vi "cno_isisubopt.vi"(0 "P":dbl[](array[numeric]), 1 "cno data":T5, 3 "tuning parameters":T1={"constraint weight"=1.0, "maximum minor iterations"=10}, 5 "L":dbl[](array[numeric]), 7 "H":dbl[][](array[numeric]), 9 "OB":dbl[](array[numeric]), 11 "error in (no error)":errorcluster, 12 "PB":dbl[][](array[numeric]), 14 "user defined functions":T2) -> (4 "P":dbl[](array[numeric]), 6 "L":dbl[](array[numeric]), 8 "H":dbl[][](array[numeric]), 10 "number of function calls":i32, 15 "error out":errorcluster)   [LabVIEW 2014, in "NI_Gmath.lvlib"]
uses:
  NI_Gmath.lvlib
  cno_data.ctl
  cno_user defined functions.ctl
  cno_user objective function ref.ctl
  objective function data.ctl
  cno_tuning parameters.ctl
  fpuIEEE64_finiteDiffConstants.ctl
  Real Outer Product.vi
  Real Cholesky Factorization.vi
  A x Vector.vi
  Real A x B.vi
  Full Cholesky Factorization.vi
  Full Real Matrix Cholesky Factorization.vi
  Create Special Real Matrix.vi
  Matrix To Array - RM.vi
  Real Inverse Matrix.vi
  Matrix left divisionMV.vi
  NI_AALBase.lvlib
  NI_AALPro.lvlib
  NI_Matrix.lvlib
panel:
  out "B":dbl[](array[numeric])
  out "G":dbl[](array[numeric])
  out "A":dbl[][](array[numeric])
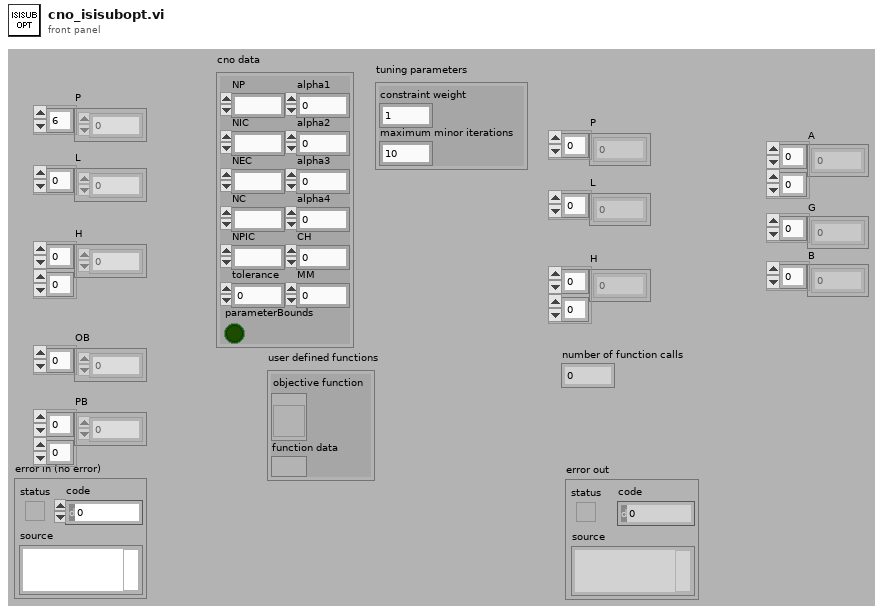
[diagram p1: front panel]
types:
  T1 = typedef "NI_Gmath.lvlib/cno_tuning parameters.ctl" = cluster{"constraint weight":dbl, "maximum minor iterations":i32}
  T2 = typedef "NI_Gmath.lvlib/cno_user defined functions.ctl" = cluster{"objective function":T3, "function data":T4}
  T3 = typedef "NI_Gmath.lvlib/cno_user objective function ref.ctl" = refnum<vi>
  T4 = typedef "NI_Gmath.lvlib/objective function data.ctl" = variant
  T5 = typedef "NI_Gmath.lvlib/cno_data.ctl" = cluster{"NP":i32, "NIC":i32, "NEC":i32, "NC":i32, "NPIC":i32, "parameterBounds":bool, "alpha1":dbl, "alpha2":dbl, "alpha3":dbl, "alpha4":dbl, "CH":i32, "MM":i32, "tolerance":dbl}
  T6 = enum32{"General", "Positive Definite", "Lower Triangular", "Upper Triangular"}
  T7 = enum32{"Identity", "Diagonal", "Toepliz", "Vandermonde", "Companion"}
  T8 = typedef "NI_Gmath.lvlib/fpuIEEE64_finiteDiffConstants.ctl" = dbl
  T9 = typedef "NI_Matrix.lvlib/RealMatrix.ctl" = dbl[][]
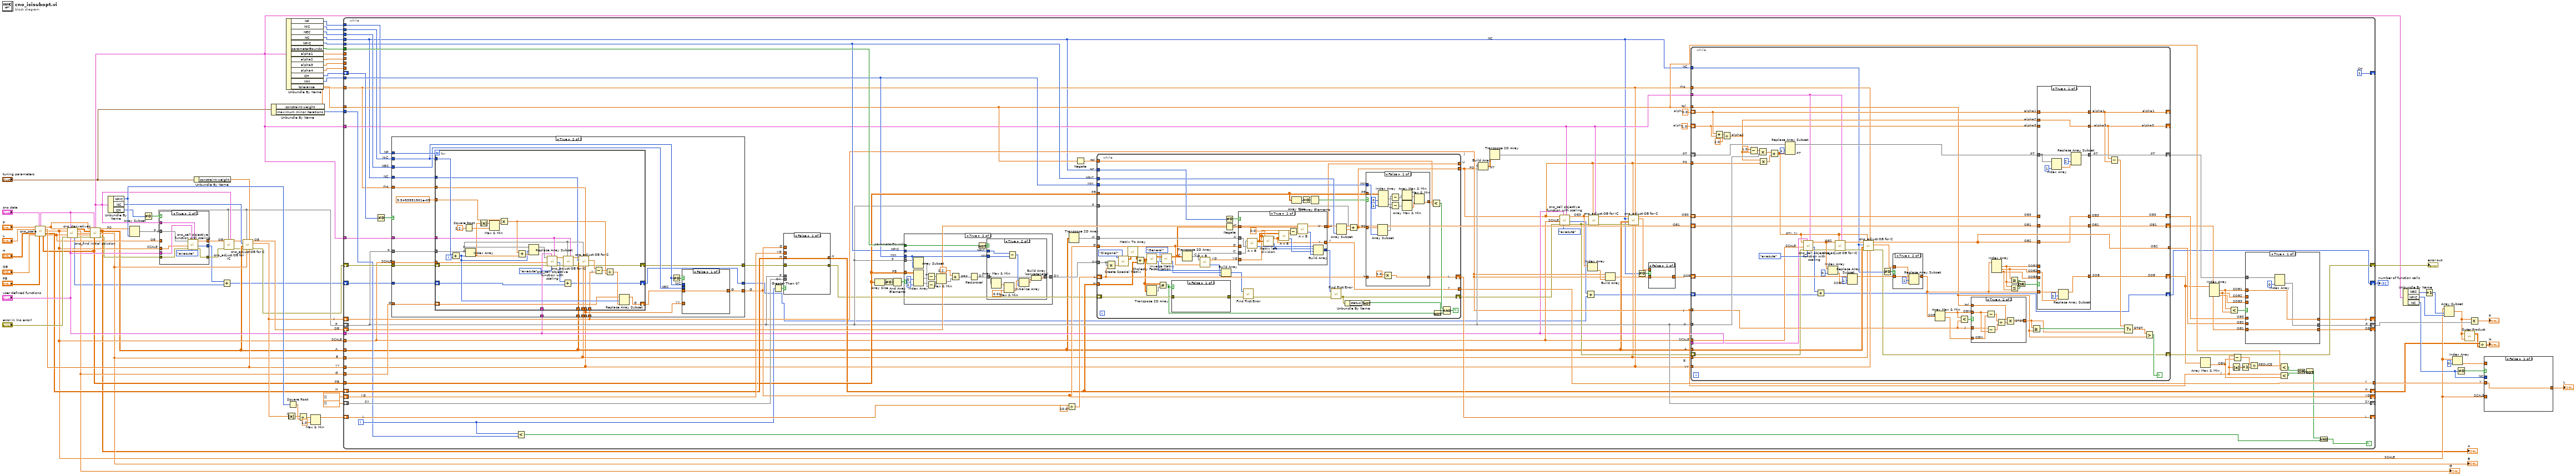
[diagram p0: block diagram]
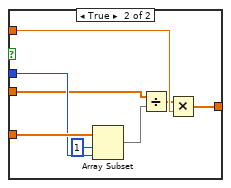
[diagram p2: hidden frame]
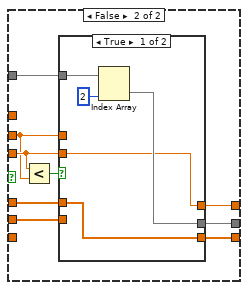
[diagram p3: hidden frame]
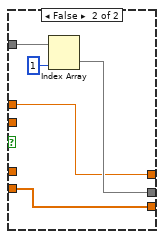
[diagram p4: hidden frame]
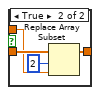
[diagram p5: hidden frame]
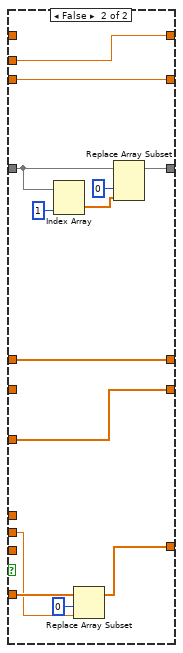
[diagram p6: hidden frame]
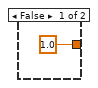
[diagram p7: hidden frame]
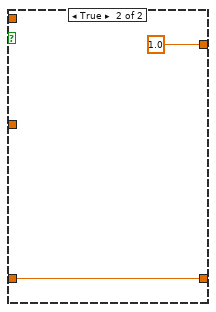
[diagram p9: hidden frame]
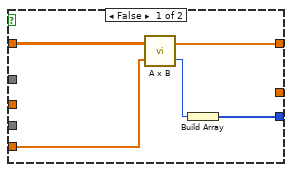
[diagram p10: hidden frame]
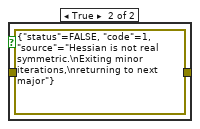
[diagram p11: hidden frame]
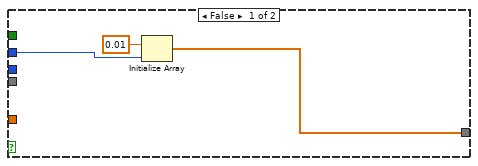
[diagram p12: hidden frame]
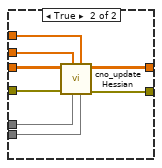
[diagram p14: hidden frame]
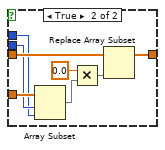
[diagram p16: hidden frame]
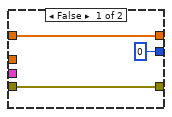
[diagram p17: hidden frame]
diagram:
  # "OB"
  # "NC"
  # "SCALE"
  # "Y"
  # "SCALE"
  # "H"
  # "OB"
  # "OB"
  # "PB"
  # "J"
  # "G"
  # "YY"
  # "B"
  # "A"
  # "SCALE"
  # "P"
  # "J"
  # "P0"
  # "P"
  # "OB"
  # "SCALE"
  n1 = call "cno_scale.vi"("P"="P", "cno data"="cno data", "L"="L", "H"="H", "OB"="OB", "PB"="PB") -> ("cno data"=w66:T5, "P"=w71:dbl[], "L"=w45:dbl[], "SCALE"=w25:dbl[], "H"=w40:dbl[][], "PB"=w43:dbl[][], "OB"=w38:dbl[])  [unwired: 3 in]
  n2 = call "cno_derivatives.vi"("P"=w71, "cno data"=w66, "SCALE"=w25, "OB"=w38, "error in (no error)"="error in (no error)", "user defined functions"="user defined functions") -> ("A"=w70:dbl[][], "G"=w37:dbl[], "B"=w69:dbl[], "CONSTRAINT"=w68:dbl[], "number of function calls"=w3:i32, "error"=w78:errorcluster)  [unwired: 4 in]
  "G" <- w37
  n3 = call "cno_find initial solution.vi"("P0"=w71, "cno data"=w66, "A"=w70, "B"=w69, "CONSTRAINT"=w68, "error"=w78, "PB"=w43) -> ("cno data"=w13:T5, "P0"=w63:dbl[], "A"=w9:dbl[][], "B"=w20:dbl[], "error"=w64:errorcluster)  [unwired: 4 in]
  "A" <- w9
  "B" <- w20
  n4 = Unbundle By Name(w13) -> ("NPIC"=w81:i32, "NC"=w79:i32, "CH"=w14:i32)
  n5 = Array Subset(array=w63, length=w81) -> (w8:dbl[])  [unwired: 1 in]
  n6 = Not Equal To 0?(x=w14) -> (x != 0?=w65:bool)
  n7 = case shown="True" w65 {
    tunnel: w8 -> [_ w93]
    tunnel: w25 -> [_ w90]
    tunnel: "user defined functions" -> [_ w91]
    tunnel: w64 -> [w84 w87]
    tunnel: [w84 w86] -> w10
    tunnel: [w83 w88] -> w12
    tunnel: w38 -> [w83 _]
    tunnel: w13 -> [_ w92]
    tunnel: [0 ("num function calls") w85] -> w4
    frame False {
    }
    frame True {
      n8 = call "cno_call objective function with scaling.vi"("cno data"=w92, "function"=enum16{"initialize", "execute"}."execute", "user defined functions"=w91, "error in (no error)"=w87, "scale"=w90, "X"=w93) -> ("error out"=w86:errorcluster, "num function calls"=w85:i32, "out"=w88:dbl[])  [unwired: 3 in]
    }
  }
  n9 = Unbundle By Name("tuning parameters") -> ("constraint weight"=w44:dbl)
  n10 = Add(x=w4, y=w3) -> (x+y=w2:i32)
  n11 = call "cno_adjust OB for IC.vi"("cno data"=w13, "P"=w8, "error in (no error)"=w10, "OB"=w12) -> ("error out"=w7:errorcluster, "OB"=w11:dbl[])  [unwired: 6 in]
  n12 = call "cno_adjust OB for C.vi"("YY"=w45, "constraint weight"=w44, "B"=w20, "P"=w8, "error in (no error)"=w7, "A"=w9, "NC"=w79, "OB"=w11) -> ("error out"=w6:errorcluster, "J"=w80:dbl, "OB"=w18:dbl[])  [unwired: 1 in]
  n13 = Unbundle By Name("tuning parameters") -> ("constraint weight"=w42:dbl, "maximum minor iterations"=w41:i32)
  n14 = Unbundle By Name(w13) -> ("NP"=w58:i32, "NIC"=w57:i32, "NEC"=w56:i32, "NC"=w54:i32, "NPIC"=w55:i32, "parameterBounds"=w53:bool, "alpha1"=w52:dbl, "alpha2"=w51:dbl, "alpha3"=w50:dbl, "alpha4"=w49:dbl, "CH"=w17:i32, "MM"=w48:i32, "tolerance"=w5:dbl)
  n15 = Absolute Value(x=w80) -> (abs(x)=w61:dbl)
  n16 = Square Root(x=w81) -> (sqrt(x)=w60:dbl)
  n17 = Divide(x=w61, y=w60) -> (x/y=w59:dbl)
  n18 = Max & Min(x=w59, y=1.0) -> (max(x,y)=w39:dbl)  [unwired: 1 out]
  n19 = while {
    tunnel: w58 -> [w137]
    tunnel: w57 -> [w157]
    tunnel: w56 -> [w156]
    tunnel: w55 -> [w155]
    tunnel: w54 -> [w101]
    tunnel: w53 -> [w174]
    tunnel: w52 -> [_]
    tunnel: w51 -> [_]
    tunnel: w50 -> [_]
    tunnel: w49 -> [_]
    tunnel: w48 -> [w167]
    tunnel: "user defined functions" -> [w112]
    tunnel: w25 -> [w113]
    tunnel: w9 -> [w105]
    tunnel: w20 -> [w104]
    tunnel: w45 -> [w103]
    tunnel: w37 -> [w183]
    shift-right: [w185] -> w19
    shift-left: w6 -> [w181]
    shift-right: [w147] -> _
    shift-left: dbl[] [] ("G") -> [w180]
    shift-right: [w148] -> _
    shift-left: dbl[] [] -> [w179]
    shift-right: [w146] -> w23
    shift-left: w40 -> [w178]
    shift-right: [w158] -> _
    shift-left: w39 -> [w173]
    tunnel: w43 -> [w168]
    tunnel: w5 -> [w125]
    shift-right: [w143] -> w33
    shift-left: w8 -> [w148]
    shift-right: [w141] -> _
    shift-left: w18 -> [w159]
    tunnel: w42 -> [w102]
    tunnel: w41 -> [w153]
    shift-right: [w145] -> _
    shift-left: w80 -> [w130]
    tunnel: [w138] -> w30
    shift-right: [1 ("CH")] -> _
    shift-left: w17 -> [w132]
    tunnel: w13 -> [w118]
    tunnel: w13 -> [w110]
    shift-right: [w94] -> w1
    shift-left: w2 -> [w98]
    i -> [w154]
    stop <- w119 continue-if-true
    # "OB"
    # "P"
    # "REDUCE"
    # "J"
    # "OBN"
    # "CH"
    # "J"
    # "Y"
    # "OB3"
    # "OB2"
    # "OB1"
    # "H"
    # "SOB3"
    # "SOB2"
    # "SOB1"
    # "tol"
    # "PT"
    # "J"
    # "rho"
    # "YY"
    # "B"
    # "A"
    # "P0"
    # "NC"
    # "G"
    # "L"
    # "alpha3"
    # "alpha1"
    # "OB3"
    # "SOB"
    # "P"
    # "SCALE"
    # "NC"
    # "OB1"
    # "OB3"
    # "SCALE"
    # "PT"
    # "J"
    # "P0"
    # "U"
    # "DX"
    # "-tol"
    # "MM"
    # "PB"
    # "NPIC"
    # "P"
    # "A'"
    # "NC"
    # "G"
    # "L"
    # "DX"
    # "parameterBounds"
    # "NPIC"
    # "MM"
    # "P"
    # "PB"
    # "L"
    # "H"
    # "P"
    # "H"
    # "H"
    # "SX"
    # "YG"
    # "SX"
    # "YG"
    # "SX"
    # "YG"
    # "G"
    # "G"
    # "rho"
    # "NEC"
    # "SCALE"
    # "P"
    # "NP"
    # "NIC"
    # "NC"
    n20 = Not Equal To 0?(x=w132) -> (x != 0?=w184:bool)
    n21 = case shown="True" w184 {
      tunnel: w137 -> [_ w474]
      tunnel: w148 -> [_ w473]
      tunnel: w157 -> [_ w462]
      tunnel: w112 -> [_ w472]
      tunnel: w113 -> [_ w471]
      tunnel: w101 -> [_ w470]
      tunnel: w156 -> [_ w460]
      tunnel: w105 -> [_ w469]
      tunnel: w104 -> [_ w468]
      tunnel: w103 -> [_ w461]
      tunnel: w102 -> [_ w467]
      tunnel: w130 -> [_ w466]
      tunnel: w183 -> [w452 w465]
      tunnel: [w452 w459] -> w147
      tunnel: w181 -> [w451 w458]
      tunnel: [w451 w457] -> w117
      tunnel: w118 -> [_ w456]
      tunnel: w98 -> [w450 w454]
      tunnel: [w450 w453] -> w96
      frame False {
      }
      frame True {
        w455 = T8 9.5493951901e-09 items=["H_FINITE_DIFF_1"=9.5493951901e-09, "H_FINITE_DIFF_2"=3.2057501263e-06, "H_FINITE_DIFF_4"=0.00033989331283, "H_FINITE_DIFF_K_1"=2.8120287999e-06, "H_FINITE_DIFF_K_2"=9.1341513557e-05, "H_FINITE_DIFF_K_3"=0.00045180790895, "H_FINITE_DIFF_K_4"=0.0014917421406] ("fpuIEEE64")
        # "G"
        # "NIC"
        # "NEC"
        # "YY"
        n22 = for {
          N: w474 -> [_]
          tunnel: w473 -> [w502]
          tunnel: w462 -> [w512]
          tunnel: w472 -> [w508]
          shift-right: [w494] -> w457
          shift-left: w458 -> [w507]
          tunnel: w471 -> [w509]
          tunnel: w470 -> [w501]
          tunnel: w469 -> [w500]
          tunnel: w468 -> [w499]
          tunnel: w461 -> [w498]
          tunnel: w467 -> [w503]
          tunnel: w466 -> [w517]
          shift-right: [w514] -> w463
          shift-left: w465 -> [w513]
          tunnel: w456 -> [w506]
          tunnel: w455 -> [w490]
          shift-right: [w484] -> w453
          shift-left: w454 -> [w485]
          i -> [w520]
          # "G"
          # "J"
          n23 = Add(x=w512, y=w520) -> (x+y=w518:i32)
          n24 = Square Root(x=2.220446049250313e-16) -> (sqrt(x)=w487:dbl)
          n25 = Index Array(array=w502, index=w518) -> (element=w492:dbl)
          n26 = Absolute Value(x=w492) -> (abs(x)=w493:dbl)
          n27 = Max & Min(x=w493, y=w487) -> (max(x,y)=w491:dbl)  [unwired: 1 out]
          n28 = Multiply(x=w490, y=w491) -> (x*y=w489:T8)
          n29 = Add(x=w489, y=w492) -> (x+y=w519:T8)
          n30 = Replace Array Subset(array=w502, new element=w519, index=w518) -> (w511:dbl[])
          n31 = call "cno_call objective function with scaling.vi"("cno data"=w506, "function"=enum16{"initialize", "execute"}."execute", "user defined functions"=w508, "error in (no error)"=w507, "scale"=w509, "X"=w511) -> ("error out"=w495:errorcluster, "num function calls"=w486:i32, "out"=w505:dbl[])  [unwired: 3 in]
          n32 = Add(x=w486, y=w485) -> (x+y=w484:i32)
          n33 = call "cno_adjust OB for IC.vi"("cno data"=w506, "P"=w502, "error in (no error)"=w495, "OB"=w505) -> ("error out"=w496:errorcluster, "OB"=w504:dbl[])  [unwired: 6 in]
          n34 = call "cno_adjust OB for C.vi"("YY"=w498, "constraint weight"=w503, "B"=w499, "P"=w502, "error in (no error)"=w496, "A"=w500, "NC"=w501, "OB"=w504) -> ("error out"=w494:errorcluster, "J"=w497:dbl)  [unwired: 1 in, 1 out]
          n35 = Subtract(x=w497, y=w517) -> (x-y=w516:dbl)
          n36 = Divide(x=w516, y=w489) -> (x/y=w515:T8)
          n37 = Replace Array Subset(array=w513, new element=w515, index=w518) -> (w514:dbl[])
        }
        n38 = Not Equal To 0?(x=w462) -> (x != 0?=w464:bool)
        n39 = case shown="False" w464 {
          tunnel: w463 -> [w475 w483]
          tunnel: w462 -> [_ w480]
          tunnel: w461 -> [_ w482]
          tunnel: w460 -> [_ w481]
          tunnel: [w475 w476] -> w459
          frame False {
          }
          frame True {
            n40 = Array Subset(array=w482, index=w481, length=w480) -> (w479:dbl[])
            n41 = Multiply(x=0.0, y=w479) -> (x*y=w477:dbl[])
            n42 = Replace Array Subset(array=w483, new element=w477) -> (w476:dbl[])  [unwired: 1 in]
          }
        }
      }
    }
    n43 = Less?(x=w154, y=w153) -> (x < y?=w120:bool)
    n44 = Greater Than 0?(x=w154) -> (x > 0?=w182:bool)
    n45 = case shown="False" w182 {
      tunnel: w180 -> [_ w444]
      tunnel: w179 -> [_ w446]
      tunnel: w147 -> [_ w445]
      tunnel: w178 -> [w441 w449]
      tunnel: [w441 w448] -> w146
      tunnel: w148 -> [_ w447]
      tunnel: w117 -> [w440 w443]
      tunnel: [w440 w442] -> w116
      frame False {
      }
      frame True {
        n46 = call "cno_update Hessian.vi"("SX"=w446, "G"=w445, "P"=w447, "YG"=w444, "error in (no error)"=w443, "H"=w449) -> ("error out"=w442:errorcluster, "H"=w448:dbl[][])  [unwired: 4 in]
      }
    }
    n47 = Array Size(array=w168) -> (size(s)=w177:i32[])
    n48 = Not Equal To 0?(x=w177) -> (x != 0?=w176:bool[])
    n49 = And Array Elements(Boolean array=w176) -> (logical AND=w175:bool)
    n50 = case shown="True" w175 {
      tunnel: w168 -> [_ w427]
      tunnel: w148 -> [_ w428]
      tunnel: w167 -> [_ w415]
      tunnel: w174 -> [_ w418]
      tunnel: w155 -> [w410 w414]
      tunnel: [w409 w413] -> w171
      frame False {
        n51 = Initialize Array(0.01 ("element"), w410) -> (w409:dbl[])
      }
      frame True {
        # "NPIC"
        # "MM"
        # "DX"
        # "gap"
        n52 = Array Subset(array=w428, length=w415) -> (w429:dbl[])  [unwired: 1 in]
        n53 = Index Array(array=w427, index (col) #1=0 ("disabled index (col)"), index (col) #2=1 ("index (col)")) -> (element #1=w424:dbl[], element #2=w423:dbl[])  [unwired: 2 in]
        n54 = Subtract(x=w429, y=w424) -> (x-y=w422:dbl[])
        n55 = Subtract(x=w423, y=w429) -> (x-y=w421:dbl[])
        n56 = Max & Min(x=w422, y=w421) -> (min(x,y)=w420:dbl[])  [unwired: 1 out]
        n57 = Add(x=2.220446049250313e-16, y=w420) -> (x+y=w419:dbl[])
        n58 = Reciprocal(x=w419) -> (1/x=w416:dbl[])
        n59 = Not(x=w418) -> (.not. x?=w417:bool)
        n60 = case shown="True" w417 {
          tunnel: w416 -> [w430 w433]
          tunnel: w415 -> [_ w435]
          tunnel: w414 -> [_ w436]
          tunnel: [w430 w431] -> w413
          frame False {
          }
          frame True {
            n61 = Array Max & Min(array=w433) -> (min value=w438:dbl)  [unwired: 3 out]
            n62 = Max & Min(x=w438, y=0.01) -> (min(x,y)=w437:dbl)  [unwired: 1 out]
            n63 = Subtract(x=w436, y=w435) -> (x-y=w434:i32)
            n64 = Initialize Array(w437, w434) -> (w432:dbl[])
            n65 = Build Array (concatenate)(w433, w432) -> (w431:dbl[])
          }
        }
      }
    }
    n66 = Divide(x=w173, y=10.0) -> (x/y=w170:dbl)
    n67 = Transpose 2D Array(2D array=w105) -> (transposed array=w169:dbl[][])
    n68 = Negate(x=w125) -> (-x=w166:dbl)
    n69 = while {
      tunnel: w171 -> [w365]
      shift-right: [w327] -> w114
      shift-left: w116 -> [w361]
      tunnel: w147 -> [w367]
      tunnel: w101 -> [w357]
      tunnel: w169 -> [w354]
      tunnel: w148 -> [w348]
      tunnel: w155 -> [w350]
      tunnel: w168 -> [w344]
      tunnel: w167 -> [w343]
      shift-right: [w341] -> w158
      shift-left: w170 -> [w342]
      tunnel: w166 -> [w339]
      tunnel: [w326] -> _
      tunnel: [w366] -> w108
      tunnel: w146 -> [w325]
      tunnel: [w323] -> w138
      stop <- w337 continue-if-true
      # "Y"
      # "Y"
      # "L"
      # "L"
      # "MM"
      # "PB"
      # "P0"
      # "U"
      # "-C"
      # "G"
      # "YG"
      # "A'"
      # "C'"
      # "C'"
      # "YG"
      # "C"
      n70 = Compound Arithmetic op=MULTIPLY(w365, w365, w342) -> (w364:dbl[])
      n71 = call-poly "Create Special Matrix.vi"("matrix type"=T7."Diagonal", "Input Vector1"=w364) -> ("Special Matrix"=w322:T9)  [unwired: 3 in, 1 out]
      n72 = call-poly "Matrix To Array.vi"("Real Matrix"=w322) -> ("Real 2D Array"=w321:dbl[][])
      n73 = Add(x=w321, y=w325) -> (x+y=w324:dbl[][])
      n74 = Transpose 2D Array(2D array=w324) -> (transposed array=w362:dbl[][])
      n75 = call-poly "Cholesky Factorization.vi"("A"=w324) -> ("Cholesky"=w359:T9, "error"=w336:i32)
      n76 = Not Equal?(x=w324, y=w362) -> (x != y?=w360:bool)
      n77 = call-poly "Inverse Matrix.vi"("matrix type"=T6."General", "Input Matrix"=w359) -> ("error"=w335:i32, "Inverse Matrix"=w352:T9)
      n78 = case shown="False" w360 {
        tunnel: w361 -> [w407 _]
        tunnel: [w407 errorcluster {"status"=FALSE, "code"=1, "source"="Hessian is not real symmetric.\nExiting minor iterations,\nreturning to next major"}] -> w332
        frame False {
        }
        frame True {
        }
      }
      n79 = Transpose 2D Array(2D array=w352) -> (transposed array=w355:T9)
      n80 = call-poly "A x B.vi"("Vector"=w367, "A"=w355) -> ("error"=w334:i32, "A x Vector"=w353:dbl[])
      n81 = Build Array(w336, w335, w334) -> (w333:i32[])
      n82 = Not Equal To 0?(x=w357) -> (x != 0?=w356:bool)
      n83 = Negate(x=w352) -> (-x=w351:T9)
      n84 = case shown="True" w356 {
        tunnel: w355 -> [_ w405]
        tunnel: w354 -> [_ w404]
        tunnel: w353 -> [w390 w402]
        tunnel: w367 -> [_ _]
        tunnel: w351 -> [w391 w400]
        tunnel: [w389 w398] -> w326
        tunnel: [w387 w397] -> w368
        tunnel: [_ w392] -> w323
        frame False {
          n85 = call-poly "A x B.vi"("Vector"=w390, "A"=w391) -> ("error"=w388:i32, "A x Vector"=w389:dbl[])
          n86 = Build Array(w388) -> (w387:i32[])
        }
        frame True {
          # "Y"
          # "U"
          # "Y"
          n87 = call-poly "A x B.vi"("B"=w404, "A"=w405) -> ("error"=w393:i32, "A x B"=w403:T9)
          n88 = call-poly "Matrix left division.vi"("A"=w402, "B"=w403, "SVD relative tolerance"=0.0) -> ("error"=w394:i32, "B\\A"=w392:dbl[])  [unwired: 1 in]
          n89 = call-poly "A x B.vi"("Vector"=w392, "A"=w403) -> ("error"=w395:i32, "A x Vector"=w401:dbl[])
          n90 = Subtract(x=w402, y=w401) -> (x-y=w399:dbl[])
          n91 = call-poly "A x B.vi"("Vector"=w399, "A"=w400) -> ("error"=w396:i32, "A x Vector"=w398:dbl[])
          n92 = Build Array(w393, w394, w395, w396) -> (w397:i32[])
        }
      }
      n93 = call "Find First Error.vi"("error in (no error)"=w332, "error codes"=w333) -> ("error out"=w331:errorcluster)  [unwired: 2 in, 1 out]
      n94 = Array Size(array=w344) -> (size(s)=w347:i32[])
      n95 = Equal To 0?(x=w347) -> (x = 0?=w346:bool[])
      n96 = Or Array Elements(Boolean array=w346) -> (logical OR=w345:bool)
      n97 = call "Find First Error.vi"("error in (no error)"=w331, "error codes"=w368) -> ("error out"=w327:errorcluster)  [unwired: 2 in, 1 out]
      n98 = Array Subset(array=w326, length=w350) -> (w349:dbl[])  [unwired: 1 in]
      n99 = Unbundle By Name(w327) -> ("status"=w330:bool)
      n100 = Add(x=w348, y=w349) -> (x+y=w366:dbl[])
      n101 = Not(x=w330) -> (.not. x?=w328:bool)
      n102 = case shown="False" w345 {
        tunnel: w366 -> [w380 _]
        tunnel: w344 -> [w381 _]
        tunnel: w343 -> [w383 _]
        tunnel: w342 -> [w378 w386]
        tunnel: [w376 w386] -> w341
        tunnel: [w371 1.0] -> w340
        frame False {
          n103 = Array Subset(array=w380, length=w383) -> (w384:dbl[])  [unwired: 1 in]
          n104 = Index Array(array=w381, index (col) #1=0 ("disabled index (col)"), index (col) #2=1 ("index (col)")) -> (element #1=w370:dbl[], element #2=w369:dbl[])  [unwired: 2 in]
          n105 = Multiply(x=2.0, y=w378) -> (x*y=w376:dbl)
          n106 = Subtract(x=w384, y=w370) -> (x-y=w374:dbl[])
          n107 = Subtract(x=w369, y=w384) -> (x-y=w375:dbl[])
          n108 = Array Max & Min(array=w374) -> (min value=w373:dbl)  [unwired: 3 out]
          n109 = Array Max & Min(array=w375) -> (min value=w372:dbl)  [unwired: 3 out]
          n110 = Max & Min(x=w373, y=w372) -> (min(x,y)=w371:dbl)  [unwired: 1 out]
        }
        frame True {
        }
      }
      n111 = Less?(x=w340, y=w339) -> (x < y?=w329:bool)
      n112 = Not(x=w360) -> (.not. x?=w338:bool)
      n113 = Compound Arithmetic op=AND(w329, w328, w338) -> (w337:bool)
    }
    n114 = Build Array(w148, w148, w108) -> (w165:dbl[][])
    n115 = Transpose 2D Array(2D array=w165) -> (transposed array=w164:dbl[][])
    n116 = call "cno_call objective function with scaling.vi"("cno data"=w110, "function"=enum16{"initialize", "execute"}."execute", "user defined functions"=w112, "error in (no error)"=w114, "scale"=w113, "X"=w108) -> ("error out"=w107:errorcluster, "num function calls"=w97:i32, "out"=w111:dbl[])  [unwired: 3 in]
    n117 = Add(x=w97, y=w96) -> (x+y=w95:i32)
    n118 = Index Array(array=w111) -> (element=w162:dbl)  [unwired: 1 in]
    n119 = call "cno_adjust OB for IC.vi"("cno data"=w110, "P"=w108, "error in (no error)"=w107, "OB"=w111) -> ("error out"=w106:errorcluster, "OB"=w109:dbl[])  [unwired: 6 in]
    n120 = Build Array(w130, w130, w162) -> (w161:dbl[])
    n121 = call "cno_adjust OB for C.vi"("YY"=w103, "constraint weight"=w102, "B"=w104, "P"=w108, "error in (no error)"=w106, "A"=w105, "NC"=w101, "OB"=w109) -> ("J"=w100:dbl, "OB"=w99:dbl[])  [unwired: 1 in, 1 out]
    n122 = Not Equal To 0?(x=w101) -> (x != 0?=w163:bool)
    n123 = case shown="False" w163 {
      tunnel: w161 -> [w210 w214]
      tunnel: [w210 w212] -> w160
      tunnel: w100 -> [_ w211]
      frame False {
      }
      frame True {
        n124 = Replace Array Subset(array=w214, new element=w211, index=2) -> (w212:dbl[])
      }
    }
    n125 = while {
      tunnel: w113 -> [w231]
      tunnel: w148 -> [w275]
      shift-right: [w243] -> w142
      shift-left: w159 -> [w246]
      tunnel: w112 -> [w232]
      tunnel: w101 -> [w226]
      tunnel: w108 -> [w274]
      shift-right: [w245] -> w144
      shift-left: w164 -> [w271]
      shift-right: [w218] -> w185
      shift-left: w107 -> [w233]
      tunnel: w105 -> [w280]
      tunnel: w104 -> [w223]
      tunnel: w103 -> [w222]
      tunnel: w102 -> [w224]
      tunnel: w130 -> [w262]
      shift-right: [w252] -> w134
      shift-left: w160 -> [w268]
      tunnel: w125 -> [w236]
      shift-right: [w244] -> w139
      shift-left: w99 -> [w247]
      shift-right: [w240] -> _
      shift-left: 0.0 -> [w251]
      shift-right: [w241] -> _
      shift-left: 1.0 -> [w249]
      tunnel: [w220] -> w140
      tunnel: w110 -> [w229]
      shift-right: [w215] -> w94
      shift-left: w95 -> [w216]
      stop <- w235 continue-if-true
      # "OB2"
      # "PT(:,2)"
      # "alpha3"
      # "alpha1"
      # "OB3"
      # "PT"
      # "OB1"
      # "gogo"
      # "alpha3"
      # "alpha1"
      # "SOB"
      # "PT"
      # "OB3"
      # "OB1"
      # "OB1"
      # "OB2"
      # "OB3"
      # "PT"
      # "alpha3"
      # "alpha2"
      # "alpha1"
      # "SOB"
      # "SOB3"
      # "SOB2"
      # "SOB1"
      # "tol"
      # "J"
      # "OBM"
      # "SOB"
      # "SOB(1)"
      # "OB2"
      # "PT"
      # "alpha2"
      # "SCALE"
      n126 = Add(x=w251, y=w249) -> (x+y=w279:dbl)
      n127 = Divide(x=w279, y=2.0) -> (x/y=w250:dbl)
      n128 = Subtract(x=1.0, y=w250) -> (x-y=w276:dbl)
      n129 = Multiply(x=w276, y=w275) -> (x*y=w273:dbl[])
      n130 = Multiply(x=w250, y=w274) -> (x*y=w272:dbl[])
      n131 = Add(x=w273, y=w272) -> (x+y=w221:dbl[])
      n132 = Replace Array Subset(array=w271, new element=w221, index (col)=1 ("disabled index (col)")) -> (w248:dbl[][])  [unwired: 1 in]
      n133 = call "cno_call objective function with scaling.vi"("cno data"=w229, "function"=enum16{"initialize", "execute"}."execute", "user defined functions"=w232, "error in (no error)"=w233, "scale"=w231, "X"=w221) -> ("error out"=w225:errorcluster, "num function calls"=w217:i32, "out"=w230:dbl[])  [unwired: 3 in]
      n134 = Add(x=w217, y=w216) -> (x+y=w215:i32)
      n135 = Index Array(array=w230, index=0) -> (element=w266:dbl)
      n136 = call "cno_adjust OB for IC.vi"("cno data"=w229, "P"=w221, "error in (no error)"=w225, "OB"=w230) -> ("error out"=w227:errorcluster, "OB"=w228:dbl[])  [unwired: 6 in]
      n137 = Replace Array Subset(array=w268, new element=w266, index=1) -> (w264:dbl[])
      n138 = call "cno_adjust OB for C.vi"("YY"=w222, "constraint weight"=w224, "B"=w223, "P"=w221, "error in (no error)"=w227, "A"=w280, "NC"=w226, "OB"=w228) -> ("error out"=w218:errorcluster, "J"=w219:dbl, "OB"=w220:dbl[])  [unwired: 1 in]
      n139 = Not Equal To 0?(x=w226) -> (x != 0?=w265:bool)
      n140 = case shown="True" w265 {
        tunnel: w264 -> [w316 w320]
        tunnel: [w316 w318] -> w259
        tunnel: w219 -> [_ w317]
        frame False {
        }
        frame True {
          n141 = Replace Array Subset(array=w320, new element=w317, index=1) -> (w318:dbl[])
        }
      }
      n142 = Array Max & Min(array=w259) -> (max value=w261:dbl, min value=w260:dbl)  [unwired: 2 out]
      n143 = Less?(x=w261, y=w262) -> (x < y?=w263:bool)
      n144 = case shown="True" w263 {
        tunnel: w262 -> [_ w314]
        tunnel: w261 -> [_ w313]
        tunnel: w260 -> [_ w315]
        tunnel: w236 -> [_ w308]
        tunnel: [1.0 w309] -> w239
        frame False {
        }
        frame True {
          # "gogo"
          # "OBN"
          n145 = Subtract(x=w313, y=w315) -> (x-y=w312:dbl)
          n146 = Subtract(x=w314, y=w313) -> (x-y=w311:dbl)
          n147 = Divide(x=w312, y=w311) -> (x/y=w310:dbl)
          n148 = Multiply(x=w308, y=w310) -> (x*y=w309:dbl)
        }
      }
      n149 = Index Array(array=w259) -> (element #1=w257:dbl, element #2=w258:dbl, element #3=w256:dbl)  [unwired: 3 in]
      n150 = Greater Or Equal?(x=w258, y=w257) -> (x >= y?=w255:bool)
      n151 = Less Or Equal?(x=w257, y=w256) -> (x <= y?=w254:bool)
      n152 = Or(x=w255, y=w254) -> (x .or. y?=w253:bool)
      n153 = Greater Or Equal?(x=w239, y=w236) -> (x >= y?=w242:bool)
      n154 = case shown="True" w253 {
        tunnel: w259 -> [w293 w306]
        tunnel: w220 -> [w283 w296]
        tunnel: w257 -> [_ _]
        tunnel: w256 -> [_ _]
        tunnel: w258 -> [w291 w304]
        tunnel: [w290 w303] -> w252
        tunnel: w251 -> [w281 _]
        tunnel: w250 -> [w282 w294]
        tunnel: w249 -> [_ w302]
        tunnel: [w282 w302] -> w241
        tunnel: w248 -> [w288 w300]
        tunnel: [w285 w297] -> w245
        tunnel: w247 -> [_ w295]
        tunnel: w246 -> [w284 _]
        tunnel: [w283 w295] -> w244
        tunnel: [w284 w296] -> w243
        tunnel: [w281 w294] -> w240
        frame True {
          n155 = Index Array(array=w288, index (col)=1 ("disabled index (col)")) -> (element=w286:dbl[])  [unwired: 1 in]
          n156 = Replace Array Subset(array=w293, new element=w291, index=2) -> (w290:dbl[])
          n157 = Replace Array Subset(array=w288, new element=w286, index (col)=2 ("disabled index (col)")) -> (w285:dbl[][])  [unwired: 1 in]
        }
        frame False {
          n158 = Index Array(array=w300, index (col)=1 ("disabled index (col)")) -> (element=w298:dbl[])  [unwired: 1 in]
          n159 = Replace Array Subset(array=w306, new element=w304, index=0) -> (w303:dbl[])
          n160 = Replace Array Subset(array=w300, new element=w298, index (col)=0 ("disabled index (col)")) -> (w297:dbl[][])  [unwired: 1 in]
        }
      }
      n161 = Subtract(x=w241, y=w240) -> (x-y=w238:dbl)
      n162 = Select(t=w238, s=w242, f=w239) -> (s? t:f=w237:dbl)
      n163 = Greater?(x=w237, y=w236) -> (0:w235:bool)
    }
    n164 = Array Max & Min(array=w134) -> (min value=w131:dbl)  [unwired: 3 out]
    n165 = Index Array(array=w134) -> (element #1=w152:dbl, element #2=w151:dbl, element #3=w150:dbl)  [unwired: 3 in]
    n166 = Less?(x=w152, y=w151) -> (x < y?=w149:bool)
    n167 = Absolute Value(x=w130) -> (abs(x)=w129:dbl)
    n168 = Subtract(x=w130, y=w131) -> (x-y=w128:dbl)
    n169 = Increment(x=w129) -> (x+1=w127:dbl)
    n170 = case shown="True" w149 {
      tunnel: w152 -> [w190 _]
      tunnel: w151 -> [_ w192]
      tunnel: w150 -> [_ w196]
      tunnel: [w190 w195] -> w145
      tunnel: w144 -> [w189 w199]
      tunnel: [w188 w198] -> w143
      tunnel: w142 -> [w187 _]
      tunnel: [w187 w194] -> w141
      tunnel: w140 -> [_ w191]
      tunnel: w139 -> [_ w193]
      frame True {
        n171 = Index Array(array=w189, index (col)=0 ("disabled index (col)")) -> (element=w188:dbl[])  [unwired: 1 in]
      }
      frame False {
        n172 = Less?(x=w196, y=w192) -> (x < y?=w197:bool)
        n173 = case shown="True" w197 {
          tunnel: w199 -> [w204 w209]
          tunnel: [w202 w207] -> w198
          tunnel: w196 -> [w201 _]
          tunnel: [w201 w206] -> w195
          tunnel: [w200 w205] -> w194
          tunnel: w193 -> [w200 _]
          tunnel: w192 -> [_ w206]
          tunnel: w191 -> [_ w205]
          frame True {
            n174 = Index Array(array=w204, index (col)=2 ("disabled index (col)")) -> (element=w202:dbl[])  [unwired: 1 in]
          }
          frame False {
            n175 = Index Array(array=w209, index (col)=1 ("disabled index (col)")) -> (element=w207:dbl[])  [unwired: 1 in]
          }
        }
      }
    }
    n176 = Divide(x=w128, y=w127) -> (x/y=w126:dbl)
    n177 = Less?(x=w126, y=w125) -> (x < y?=w124:bool)
    n178 = Less?(x=w130, y=w131) -> (x < y?=w123:bool)
    n179 = Or(x=w124, y=w123) -> (x .or. y?=w122:bool)
    n180 = Not(x=w122) -> (.not. x?=w121:bool)
    n181 = And(x=w121, y=w120) -> (x .and. y?=w119:bool)
  }
  "error out" <- w19
  "number of function calls" <- w1
  n182 = Unbundle By Name(w13) -> ("NEC"=w35:i32, "NPIC"=w36:i32, "NC"=w29:i32)
  n183 = Increment(x=w35) -> (x+1=w34:i32)
  n184 = Array Subset(array=w25, index=w34, length=w36) -> (w27:dbl[])
  n185 = Index Array(array=w25, index=0) -> (element=w24:dbl)
  n186 = Not Equal To 0?(x=w29) -> (x != 0?=w31:bool)
  n187 = call-poly "Outer Product.vi"("Y Vector"=w27, "X Vector"=w27) -> ("Outer Product"=w22:T9)  [unwired: 1 out]
  n188 = Multiply(x=w27, y=w33) -> (x*y=→"P":dbl[])
  n189 = Divide(x=w23, y=w22) -> (x/y=→"H":T9)
  n190 = case shown="False" w31 {
    tunnel: w30 -> [w521 w525]
    tunnel: w25 -> [_ w528]
    tunnel: w29 -> [_ w526]
    tunnel: [w521 w522] -> w28
    tunnel: w24 -> [_ w529]
    frame False {
    }
    frame True {
      n191 = Array Subset(array=w528, index=1, length=w526) -> (w524:dbl[])
      n192 = Divide(x=w525, y=w524) -> (x/y=w523:dbl[])
      n193 = Multiply(x=w523, y=w529) -> (x*y=w522:dbl[])
    }
  }
  "L" <- w28
